vi "NXTMMX-Dual.vi"() -> ()   [LabVIEW 2009]
uses:
  <vilib>/NXT/Subs/LVHSConnector.ctl
  <vilib>/NXT/Block Support/NXT_InputPort.ctl
  mindsensors.com LVEE Toolkit/Dual/NXTMMX-DM.vi
panel:
  in  "Input Port":T1 items=["Port 1", "Port 2", "Port 3", "Port 4"]
  out "NXT dup":T2={"error"={"status"=FALSE, "code"=0, "source"=""}, "address"="", "NXT #"=-1, "Show Error"=TRUE, "Connection"=4} {"Connection" items=["USB", "Bluetooth", "USB then Bluetooth", "Last Connection", "Preference"]}
  in  "NXT":T2={"error"={"status"=FALSE, "code"=0, "source"=""}, "address"="", "NXT #"=-1, "Show Error"=TRUE, "Connection"=4} {"Connection" items=["USB", "Bluetooth", "USB then Bluetooth", "Last Connection", "Preference"]}
  in  "Input of Motor Multiplexer":T3={"NXTMMX Address"=6, "Which Motor"=0, "Operation"=0, "Next Action"=0, "Position"=0, "Direction"=FALSE, "Power"=100, "Durartion"=0, "Wait for Completion"=FALSE, "Relative"=FALSE} {"Next Action" items=["Float", "Brake"]; "Operation" items=["Run Unlimited", "Run Seconds", "Run Tachometer"]; "Which Motor" items=["Motor 1", "Motor 2", "Both Motors"]; "NXTMMX Address" min=2 max=254 step=2 format="%x"}
  out "Output of Motor Multiplexer":T4
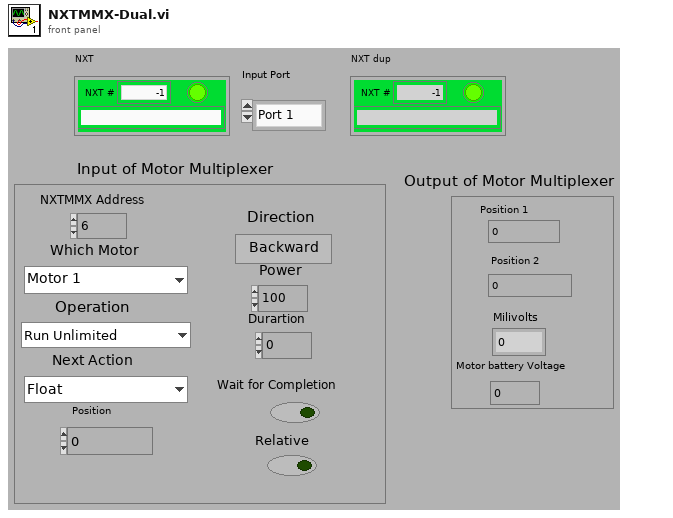
[diagram p1: front panel]
types:
  T1 = typedef "NXT_InputPort.ctl" = u8
  T2 = typedef "LVHSConnector.ctl" = cluster{"error":errorcluster, "address":string, "NXT #":i32, "Show Error":bool, "Connection":u16}
  T3 = cluster{"NXTMMX Address":u8, "Which Motor":u8, "Operation":u8, "Next Action":u8, "Position":i32, "Direction":bool, "Power":i8, "Durartion":u8, "Wait for Completion":bool, "Relative":bool}
  T4 = cluster{"Milivolts":u16, "Position 1":i32, "Position 2":i32, "Motor battery Voltage":dbl}
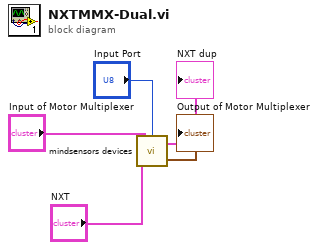
[diagram p0: block diagram]
diagram:
  n1 = call-poly "mindsensors devices.vi"("Input of Motor Multiplexer"="Input of Motor Multiplexer", "NXT"="NXT", "Input Port"="Input Port") -> ("Output of Motor Multiplexer"=→"Output of Motor Multiplexer":T4, "NXT dup"=→"NXT dup":T2)
